vi "Add Columns.vi"(8 "error in":errorcluster, 10 "Sheet Name":string, 11 "SpreadsheetDoc in":refnum<k24>) -> (0 "error out":errorcluster, 2 "Columns":refnum<k24>, 3 "SpreadsheetDoc out":refnum<k24>)   [LabVIEW 2019, in "Open Xml.lvlib"]
uses:
  Open Xml.lvlib
  D:/git/Open-Xml-LabVIEW/Source/DocumentFormat.OpenXml.dll
  DocumentFormat.OpenXml.dll
  D:/git/Open-Xml-LabVIEW/Source/OpenXmlGenericsWrapper.dll
  OpenXmlGenericsWrapper.dll
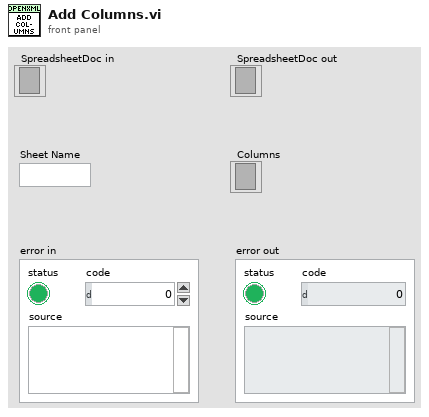
[diagram p1: front panel]
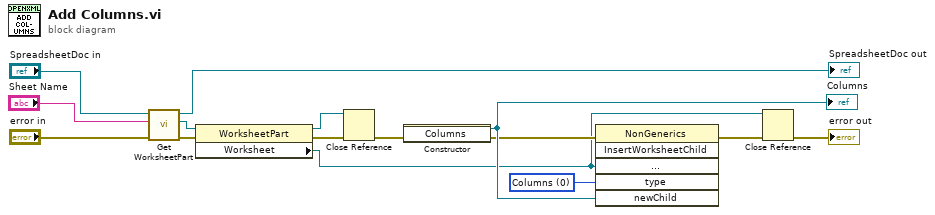
[diagram p0: block diagram]
diagram:
  w11 = 0 items=["Columns", "SheetViews", "SheetFormatPr", "PageMargins", "PageSetup", "HeaderFooter", "ConditionalFormatting", "DataValidations", "MergeCells", "Hyperlinks", "Drawing", "ExtLst"] ("type")
  n1 = call "Get WorksheetPart.vi"("error in"="error in", "Sheet Name"="Sheet Name", "SpreadsheetDoc in"="SpreadsheetDoc in") -> ("error out"=w5:errorcluster, "WorksheetPart"=w9:refnum<k24>, "SpreadsheetDoc out"=→"SpreadsheetDoc out":refnum<k24>)  [unwired: 5 in, 1 out]
  n2 = property class="WorksheetPart"(reference=w9, error in=w5) -> (reference out=w13:refnum<k24>, error out=w14:errorcluster, "Worksheet"=w1:refnum<k24>)
  n3 = Close Reference(reference=w13, error in (no error)=w14) -> (error out=w15:errorcluster)
  n4 = constructor class="Columns"(error in=w15) -> (reference out=w12:refnum<k24>, error out=w4:errorcluster)  [unwired: 2 in, 1 out]
  "Columns" <- w12
  n5 = invoke class="NonGenerics" method="InsertWorksheetChild"(error in=w4, "worksheet"=w1, "type"=w11, "newChild"=w12) -> (error out=w10:errorcluster)  [unwired: 2 in, 5 out]
  n6 = Close Reference(reference=w1, error in (no error)=w10) -> (error out=→"error out":errorcluster)
